vi "ConvertPlungerStatusCluster.vi"(11 "Cluster 2":T1) -> (1 "plunger status":enum16{"ASSERTED", "DE-ASSERTED\nOUT OF BEAM"}[](array[ring]), 2 "read switches":enum16{"OUT of Beam", "IN Beam", ""}[](array[ring]), 3 "Cluster 3":T1)   [LabVIEW 2011]
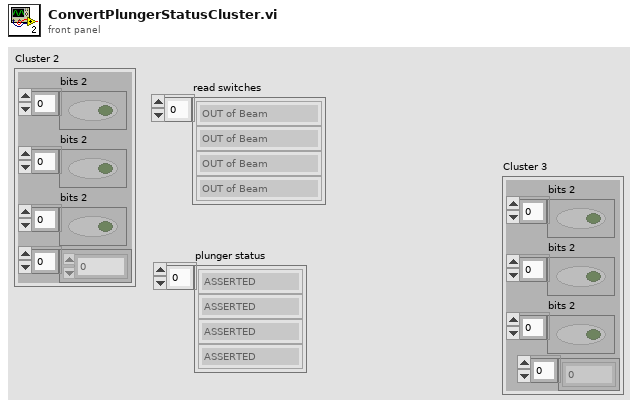
[diagram p1: front panel]
types:
  T1 = cluster{"bits 2":bool[], "bits 2":bool[], "bits 2":bool[], i32[]}
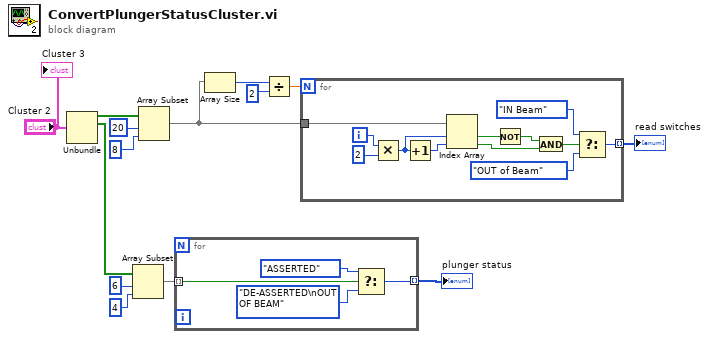
[diagram p0: block diagram]
diagram:
  n1 = Unbundle("Cluster 2") -> ("bits 2"=w14:bool[], "bits 2"=w2:bool[])  [unwired: 2 out]
  n2 = Array Subset(array=w2, index=6, length=4) -> (w1:bool[])
  n3 = Array Subset(array=w14, index=20, length=8) -> (w12:bool[])
  n4 = for {
    tunnel: [w16] -> w3 mode=indexing
    tunnel: w1 -> [w15] mode=indexing
    n5 = Select(t=enum16{"ASSERTED", "DE-ASSERTED\nOUT OF BEAM"}."ASSERTED", s=w15, f=enum16{"ASSERTED", "DE-ASSERTED\nOUT OF BEAM"}."DE-ASSERTED\nOUT OF BEAM") -> (s? t:f=w16:enum16{"ASSERTED", "DE-ASSERTED\nOUT OF BEAM"})
  }
  "plunger status" <- w3
  n6 = Array Size(array=w12) -> (size(s)=w9:i32)
  n7 = Divide(x=w9, y=2) -> (x/y=w7:dbl)
  n8 = for {
    N: w7 -> [_]
    tunnel: w12 -> [w29]
    tunnel: [w22] -> w11 mode=indexing
    i -> [w21]
    n9 = Multiply(x=w21, y=2) -> (x*y=w19:i32)
    n10 = Increment(x=w19) -> (x+1=w28:i32)
    n11 = Index Array(array=w29, index #1=w19, index #2=w28) -> (element #1=w27:bool, element #2=w26:bool)
    n12 = Not(x=w27) -> (.not. x?=w30:bool)
    n13 = And(x=w30, y=w26) -> (x .and. y?=w25:bool)
    n14 = Select(t=enum16{"OUT of Beam", "IN Beam", ""}."IN Beam", s=w25, f=enum16{"OUT of Beam", "IN Beam", ""}."OUT of Beam") -> (s? t:f=w22:enum16{"OUT of Beam", "IN Beam", ""})
  }
  "read switches" <- w11
  "Cluster 3" <- "Cluster 2"
